vi "Array_Resize 2D Array (Variant).vi"(6 "Data type (Array's single element / default values)":variant, 8 "Error In":errorcluster, 9 "Required columns":i32=1, 10 "Required rows":i32, 11 "Array to resize":variant[][](array[variant])) -> (0 "Error Out (no error)":errorcluster, 3 "Resized array":variant[][](array[variant]))   [LabVIEW 2013]
doc: "Use this VI to resize any array to the specified size.\nIf the input array is longer than the specified size it some of its last elements are eliminated.\nIf it is shorter, then elements are added to achieve the required size. The added elements will have the value you specify in the Data Type input."
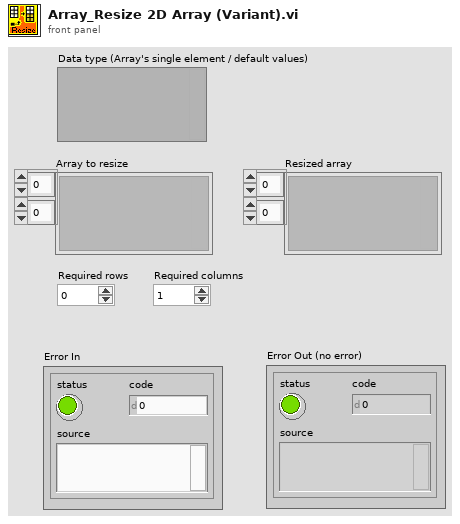
[diagram p1: front panel]
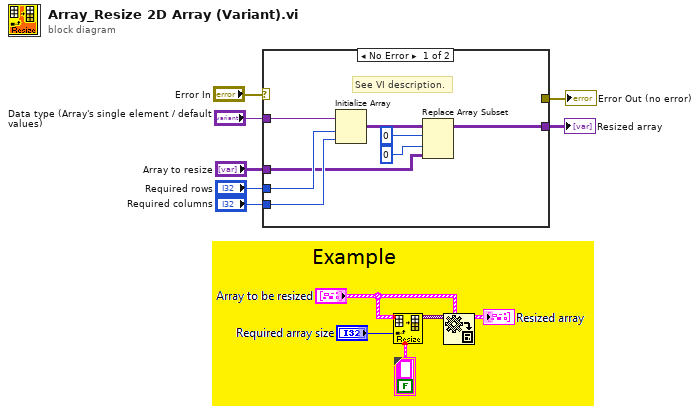
[diagram p0: block diagram]
diagram:
  n1 = case shown="No Error" "Error In" {
    selector: "Error In" -> [_ w16]
    tunnel: [w15 w17] -> w7
    tunnel: "Array to resize" -> [w10 w17]
    tunnel: "Data type (Array's single element / default values)" -> [w14 _]
    tunnel: "Required rows" -> [w13 _]
    tunnel: [_ w16] -> w2
    tunnel: "Required columns" -> [w11 _]
    frame No Error {
      # "See VI description."
      n2 = Initialize Array(w14, w13, w11) -> (w12:variant[][])
      n3 = Replace Array Subset "Replace Array Subset"(array=w12, new element=w10, index (row)=0 ("disabled index (row)"), index (col)=0 ("disabled index (col)")) -> (w15:variant[][])
    }
    frame Error {
    }
  }
  "Resized array" <- w7
  "Error Out (no error)" <- w2
